vi "1553B_CMD_Sync.vi"(11 "数据字数组":u16[](array[numeric])) -> (3 "1553B指令":string)   [LabVIEW 2012]
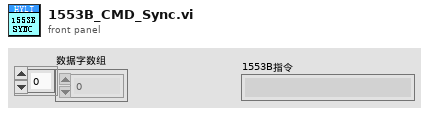
[diagram p1: front panel]
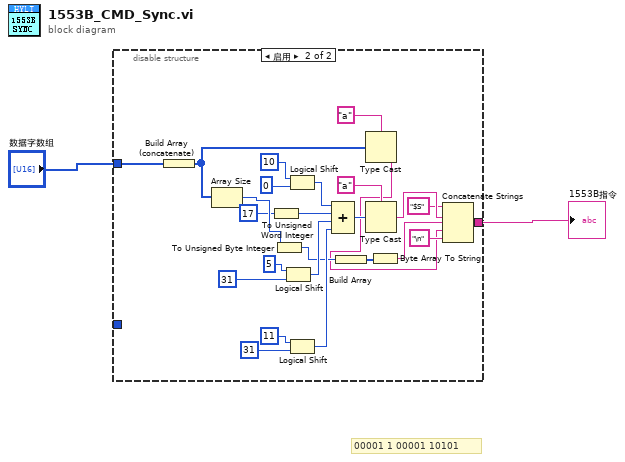
[diagram p0: block diagram]
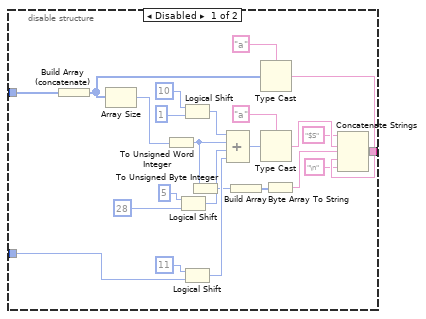
[diagram p2: hidden frame]
diagram:
  # "00001 1 00001 10101"
  n1 = disable-structure shown="启用" {
    disable-tunnel: _ -> [w19 _]
    disable-tunnel: [w10 w38] -> w2
    disable-tunnel: "数据字数组" -> [w9 w37]
    frame Disabled {
      n2 = Build Array (concatenate)(w9) -> (w8:u16[])
      n3 = Array Size(array=w8) -> (size(s)=w16:i32)
      n4 = To Unsigned Word Integer(number=w16) -> (unsigned 16bit integer=w7:u16)
      n5 = Logical Shift(y=i16 5, x=i16 28) -> (x << y=w22:i16)
      n6 = Logical Shift(y=i16 10, x=u16 1) -> (x << y=w23:u16)
      n7 = Logical Shift(y=i16 11, x=w19) -> (x << y=w18:i16)
      n8 = To Unsigned Byte Integer(number=w7) -> (unsigned 8bit integer=w5:u8)
      n9 = Compound Arithmetic op=ADD(w23, w7, w22, w18) -> (w17:u16)
      n10 = Build Array(w5) -> (w6:u8[])
      n11 = Type Cast(type="a" ("类型"), x=w8) -> (*(type *) &x=w14:string)
      n12 = Type Cast(type="a" ("类型"), x=w17) -> (*(type *) &x=w13:string)
      n13 = Byte Array To String(unsigned byte array=w6) -> (string=w4:string)
      n14 = Concatenate Strings("$S" ("字符串"), w13, w4, w14, "\n" ("字符串")) -> (w10:string)
    }
    frame Enabled {
      n15 = Build Array (concatenate)(w37) -> (w30:u16[])
      n16 = Array Size(array=w30) -> (size(s)=w29:i32)
      n17 = To Unsigned Word Integer(number=u16 17 ("数字")) -> (unsigned 16bit integer=w36:u16)
      n18 = To Unsigned Byte Integer(number=w29) -> (unsigned 8bit integer=w34:u8)
      n19 = Logical Shift(y=i16 5, x=i16 31) -> (x << y=w47:i16)
      n20 = Logical Shift(y=i16 10, x=u16 0) -> (x << y=w48:u16)
      n21 = Logical Shift(y=i16 11, x=i16 31) -> (x << y=w44:i16)
      n22 = Compound Arithmetic op=unknown(w48, w36, w47, w44) -> (w43:u16)
      n23 = Build Array(w34) -> (w35:u8[])
      n24 = Type Cast(type="a" ("类型"), x=w30) -> (*(type *) &x=w31:string)
      n25 = Type Cast(type="a" ("类型"), x=w43) -> (*(type *) &x=w41:string)
      n26 = Byte Array To String(unsigned byte array=w35) -> (string=w33:string)
      n27 = Concatenate Strings("$S" ("字符串"), w41, w33, w31, "\n" ("字符串")) -> (w38:string)
    }
  }
  "1553B指令" <- w2
